vi "LNLS Control Encode FOFBC.vi"(8 "error in (no error)":errorcluster, 11 "PFOFBC Data":T1={"Status"=0, "Operation Mode"=enum."Manual Mode", "Horizontal Gain"=0.0, "Vertical Gain"=0.0, "Selected Reference Orbit"=0, "Selected Correction Matrix"=0, "Selected FPGA Filters"=0, "Horizontal Distortion Threshold"=0.0, "Vertical Distortion Threshold"=0.0, "Timestamp"=0.0}) -> (0 "error out":errorcluster, 2 "command body":string)   [LabVIEW 2011, in "LNLS Control VIs.lvlib"]
uses:
  LNLS Control VIs.lvlib
  Types Definitions/Type Control FOFB Configuration Out.ctl
  Types Definitions/Type Operation Mode State.ctl
  Type Definitions.lvlib
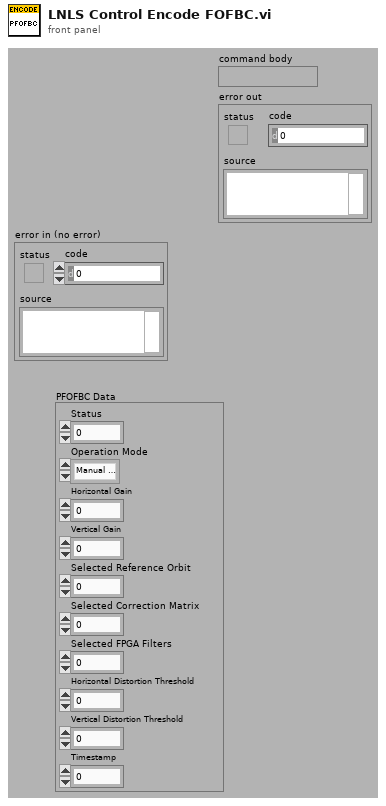
[diagram p1: front panel]
types:
  T1 = typedef "Type Definitions.lvlib/Type Control FOFB Configuration Out.ctl" = cluster{"Status":u16, "Operation Mode":T2, "Horizontal Gain":sgl, "Vertical Gain":sgl, "Selected Reference Orbit":i32, "Selected Correction Matrix":i32, "Selected FPGA Filters":i32, "Horizontal Distortion Threshold":sgl, "Vertical Distortion Threshold":sgl, "Timestamp":dbl}
  T2 = typedef "Type Definitions.lvlib/Type Operation Mode State.ctl" = enum8{"Idle Mode", "Manual Mode", "FOFB Mode"}
  T3 = enum16{"big-endian, network order", "native, host order", "little-endian"}
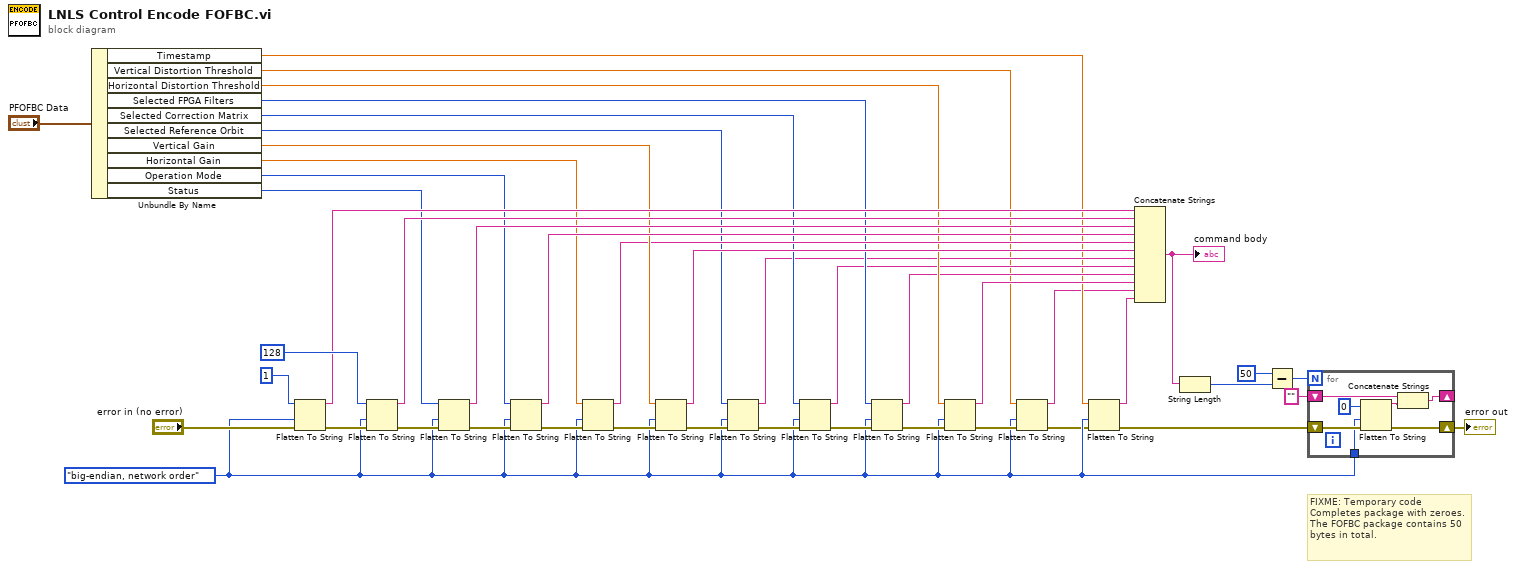
[diagram p0: block diagram]
diagram:
  w9 = T3."big-endian, network order" ("byte order (0:big-endian, network order)")
  # "FIXME: Temporary code\nCompletes package with zeroes. The FOFBC package contains 50 bytes in total."
  n1 = Unbundle By Name("PFOFBC Data") -> ("Timestamp"=w12:dbl, "Vertical Distortion Threshold"=w10:sgl, "Horizontal Distortion Threshold"=w22:sgl, "Selected FPGA Filters"=w23:i32, "Selected Correction Matrix"=w24:i32, "Selected Reference Orbit"=w25:i32, "Vertical Gain"=w30:sgl, "Horizontal Gain"=w31:sgl, "Operation Mode"=w27:T2, "Status"=w26:u16)
  n2 = Flatten To String(anything=u8 1 ("priority"), byte order (0:big-endian, network order)=w9, error in (no error)="error in (no error)") -> (data string=w38:string, error out=w40:errorcluster)  [unwired: 1 in, 1 out]
  n3 = Flatten To String(anything=u8 128 ("flag"), byte order (0:big-endian, network order)=w9, error in (no error)=w40) -> (data string=w39:string, error out=w35:errorcluster)  [unwired: 1 in, 1 out]
  n4 = Flatten To String(anything=w26, byte order (0:big-endian, network order)=w9, error in (no error)=w35) -> (data string=w33:string, error out=w45:errorcluster)  [unwired: 1 in, 1 out]
  n5 = Flatten To String(anything=w27, byte order (0:big-endian, network order)=w9, error in (no error)=w45) -> (data string=w32:string, error out=w34:errorcluster)  [unwired: 1 in, 1 out]
  n6 = Flatten To String(anything=w31, byte order (0:big-endian, network order)=w9, error in (no error)=w34) -> (data string=w29:string, error out=w44:errorcluster)  [unwired: 1 in, 1 out]
  n7 = Flatten To String(anything=w30, byte order (0:big-endian, network order)=w9, error in (no error)=w44) -> (data string=w28:string, error out=w21:errorcluster)  [unwired: 1 in, 1 out]
  n8 = Flatten To String(anything=w25, byte order (0:big-endian, network order)=w9, error in (no error)=w21) -> (data string=w17:string, error out=w20:errorcluster)  [unwired: 1 in, 1 out]
  n9 = Flatten To String(anything=w24, byte order (0:big-endian, network order)=w9, error in (no error)=w20) -> (data string=w16:string, error out=w19:errorcluster)  [unwired: 1 in, 1 out]
  n10 = Flatten To String(anything=w23, byte order (0:big-endian, network order)=w9, error in (no error)=w19) -> (data string=w15:string, error out=w18:errorcluster)  [unwired: 1 in, 1 out]
  n11 = Flatten To String(anything=w22, byte order (0:big-endian, network order)=w9, error in (no error)=w18) -> (data string=w14:string, error out=w11:errorcluster)  [unwired: 1 in, 1 out]
  n12 = Flatten To String(anything=w10, byte order (0:big-endian, network order)=w9, error in (no error)=w11) -> (data string=w8:string, error out=w1:errorcluster)  [unwired: 1 in, 1 out]
  n13 = Flatten To String(anything=w12, byte order (0:big-endian, network order)=w9, error in (no error)=w1) -> (data string=w7:string, error out=w13:errorcluster)  [unwired: 1 in, 1 out]
  n14 = Concatenate Strings(w38, w39, w33, w32, w29, w28, w17, w16, w15, w14, w8, w7) -> (w2:string)
  "command body" <- w2
  n15 = String Length(string=w2) -> (length=w5:i32)
  n16 = Subtract(x=50, y=w5) -> (x-y=w3:i32)
  n17 = for {
    N: w3 -> [_]
    shift-right: [w51] -> w37
    shift-left: w13 -> [w52]
    shift-right: [w49] -> _
    shift-left: "" -> [w48]
    tunnel: w9 -> [w46]
    n18 = Flatten To String(anything=u8 0 ("Correction Period (usec)"), byte order (0:big-endian, network order)=w46, error in (no error)=w52) -> (data string=w50:string, error out=w51:errorcluster)  [unwired: 1 in, 1 out]
    n19 = Concatenate Strings(w48, w50) -> (w49:string)
  }
  "error out" <- w37
